vi "robot_data_subscriber.vi"() -> (3 "Read Sample":T1)   [LabVIEW 2024]
uses:
  <vilib>/RTI DDS Toolkit/Types/RTI DDS Advanced Reader Configuration.ctl
  <vilib>/RTI DDS Toolkit/Types/DDS Sample Info.ctl
  <vilib>/RTI DDS Toolkit/Types/DDS Duration.ctl
  <vilib>/RTI DDS Toolkit/Types/RTI DDS Read Mode.ctl
  <vilib>/RTI DDS Toolkit/Library/LVDDS_library.lvlib
panel:
  out "DDS Sample Info":T2
  out "Timeout":bool
  in  "Advanced Reader Configuration":T3={"typeName"="octa_ros::msg::dds_::Robotdata_", "keyName"="", "domainParticipantQoSProfile"="", "dataReaderQoSProfile"="", "forceArrayMapping?"=FALSE, "forceExclusiveReader?"=FALSE, "forceRead? (only ExclusiveReader)"=FALSE, "forceUnboundedString?"=FALSE}
  # "Source Timestamp"
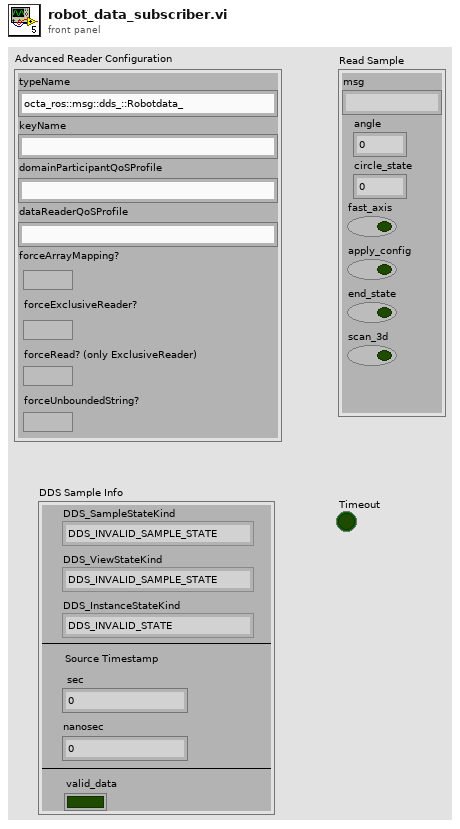
[diagram p1: front panel]
types:
  T1 = cluster{"msg":string, "angle":dbl, "circle_state":i32, "fast_axis":bool, "apply_config":bool, "end_state":bool, "scan_3d":bool}
  T2 = typedef "LVDDS_library.lvlib/DDS Sample Info.ctl" = cluster{"DDS_SampleStateKind":enum32{"DDS_INVALID_SAMPLE_STATE", "DDS_READ_SAMPLE_STATE", "DDS_NOT_READ_SAMPLE_STATE"}, "DDS_ViewStateKind":enum32{"DDS_INVALID_SAMPLE_STATE", "DDS_NEW_VIEW_STATE", "DDS_NOT_NEW_VIEW_STATE"}, "DDS_InstanceStateKind":enum32{"DDS_INVALID_STATE", "DDS_ALIVE_INSTANCE_STATE", "DDS_NOT_ALIVE_DISPOSED_INSTANCE_STATE", "", "DDS_NOT_ALIVE_NO_WRITERS_INSTANCE_STATE"}, "sec":i32, "nanosec":u32, "valid_data":bool}
  T3 = typedef "LVDDS_library.lvlib/RTI DDS Advanced Reader Configuration.ctl" = cluster{"typeName":string, "keyName":string, "domainParticipantQoSProfile":string, "dataReaderQoSProfile":string, "forceArrayMapping?":bool, "forceExclusiveReader?":bool, "forceRead? (only ExclusiveReader)":bool, "forceUnboundedString?":bool}
  T4 = typedef "LVDDS_library.lvlib/RTI DDS Read Mode.ctl" = enum32{"LVDDS_READ_MODE_POLLING", "LVDDS_READ_MODE_BLOCKING"}
  T5 = typedef "LVDDS_library.lvlib/DDS Duration.ctl" = cluster{"sec":i32, "nanosec":u32}
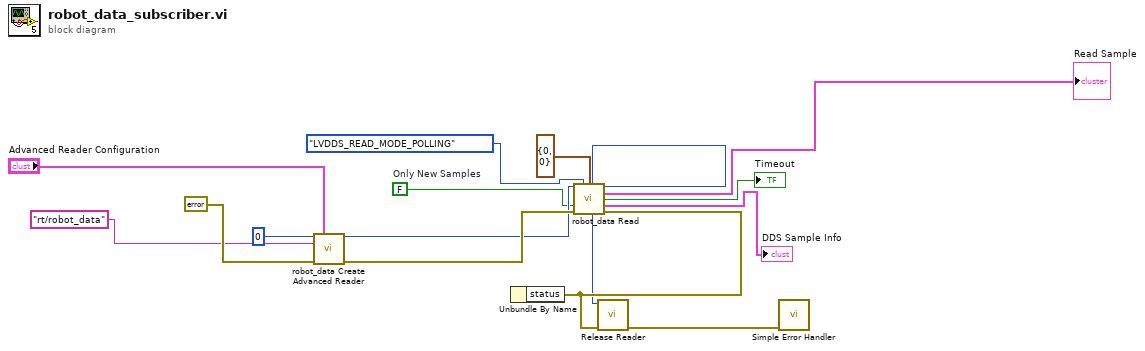
[diagram p0: block diagram]
diagram:
  w7 = FALSE  # Only New Samples
  n1 = call "robot_data Create Advanced Reader.vi"("Domain Id"=u32 0, "Advanced Reader Configuration"="Advanced Reader Configuration", "Topic Name"="rt/robot_data", "error in (no error)"=errorcluster {"status"=FALSE, "code"=0, "source"=""}) -> ("DDS Object Ref"=w10:u64, "error out"=w11:errorcluster)  [unwired: 10 in]
  n2 = call "robot_data Read.vi"("DDS Object Ref in"=w10, "Read Mode"=RTI_DDS_Read_Mode."LVDDS_READ_MODE_POLLING" ("LVDDS_Read_Mode"), "Blocking Timeout"=T5 {"sec"=0, "nanosec"=0}, "Only New Samples"=w7, "error in (no error)"=w11) -> ("DDS Object Ref out"=w12:u64, "Read Sample"=→"Read Sample":T1, "Timeout"=→"Timeout":bool, "DDS Sample Info"=→"DDS Sample Info":T2, "error out"=w13:errorcluster)  [unwired: 6 in]
  n3 = Unbundle By Name(w13) -> ()  [unwired: 1 out]
  n4 = call <vilib>:"Release Reader.vi"("error in (no error)"=w13, "DDS Object Ref"=w12) -> ("error out"=w1:errorcluster)  [unwired: 9 in]
  n5 = call <vilib>:"Simple Error Handler.vi"("error in (no error)"=w1) -> ()  [unwired: 4 in, 5 out]
